vi "CreateLogFile.vi"(0 "Buffers in":T1={"Channels"=[], "PosttriggerBuffer"=refnum, "PretriggerBuffer"=refnum, "BlockSizePerChannel"=0, " logging semaphore"=refnum, "Log refnum"=refnum, "snapshotBuffer"=refnum, "logDirectory"=path "", "logPrefix"="", "decimation factor"=1, "max files"=0, "SampleRate"=0.0}, 11 "error in (no error)":errorcluster) -> (4 "Buffers out":T1={"Channels"=[], "PosttriggerBuffer"=refnum, "PretriggerBuffer"=refnum, "BlockSizePerChannel"=0, " logging semaphore"=refnum, "Log refnum"=refnum, "snapshotBuffer"=refnum, "logDirectory"=path "", "logPrefix"="", "decimation factor"=1, "max files"=0, "SampleRate"=0.0}, 15 "error out":errorcluster)   [LabVIEW 2017, in "BufferLogging.lvlib"]
uses:
  BufferLogging.lvlib
  Buffers.ctl
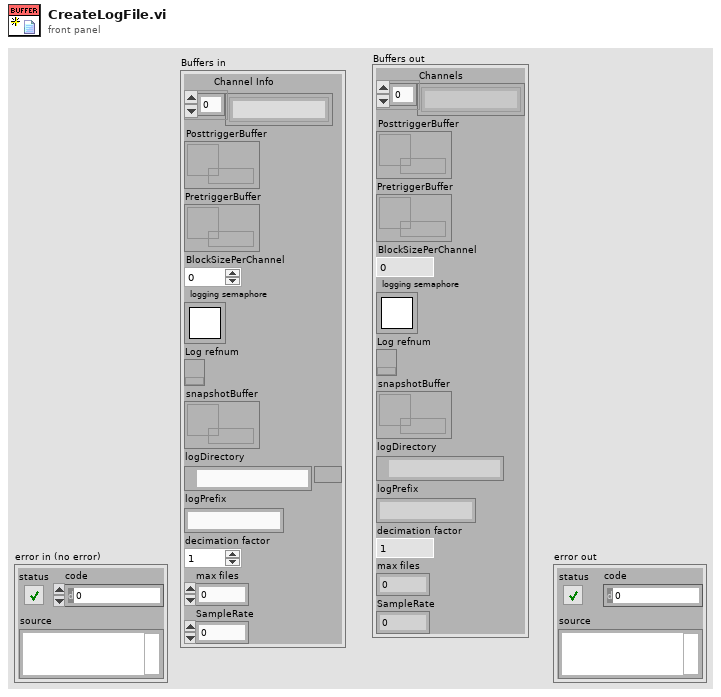
[diagram p1: front panel]
types:
  T1 = typedef "BufferLogging.lvlib/Buffers.ctl" = cluster{"Channels":string[], "PosttriggerBuffer":refnum<queue>, "PretriggerBuffer":refnum<queue>, "BlockSizePerChannel":i32, " logging semaphore":T2, "Log refnum":refnum<k34>, "snapshotBuffer":refnum<data-value>, "logDirectory":path, "logPrefix":string, "decimation factor":i32, "max files":i32, "SampleRate":dbl}
  T2 = typedef "Semaphore RefNum" = refnum<k1>
  T3 = enum16{"open", "open or create", "create or replace", "create", "open (read-only)"}
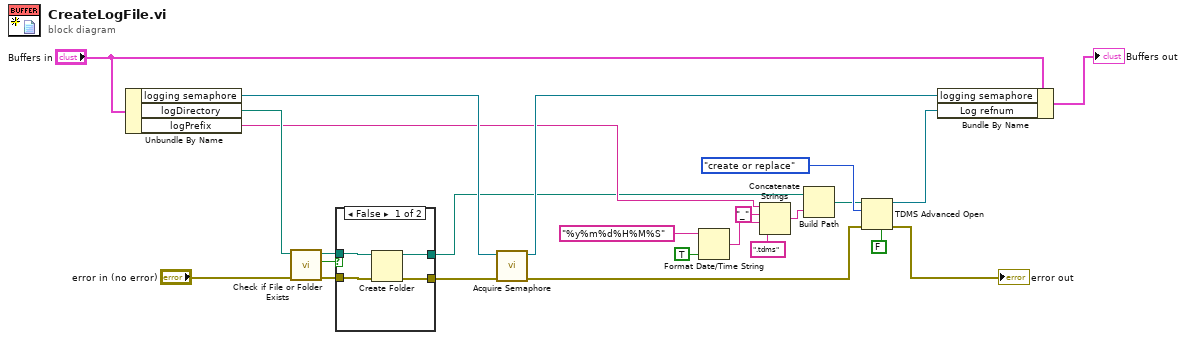
[diagram p0: block diagram]
diagram:
  n1 = Unbundle By Name("Buffers in") -> ("logging semaphore"=w15:T2, "logDirectory"=w3:path, "logPrefix"=w2:string)
  n2 = call <vilib>:"Check if File or Folder Exists.vi"("error in (no error)"="error in (no error)", "path"=w3) -> ("error out"=w6:errorcluster, "file or folder exists?"=w8:bool, "dup path"=w7:path)  [unwired: 7 in]
  n3 = case shown="False" w8 {
    tunnel: w7 -> [w27 w30]
    tunnel: w6 -> [w28 w29]
    tunnel: [w26 w30] -> w1
    tunnel: [w25 w29] -> w4
    frame False {
      n4 = Create Folder(path (use dialog)=w27, error in=w28) -> (created path=w26:path, error out=w25:errorcluster)  [unwired: 1 in, 1 out]
    }
    frame True {
    }
  }
  n5 = call <vilib>:"Acquire Semaphore.vi"("error in (no error)"=w4, "semaphore"=w15) -> ("error out"=w14:errorcluster, "semaphore out"=w12:T2)  [unwired: 3 in, 1 out]
  n6 = Format Date/Time String(time format string (%c)="%y%m%d%H%M%S", UTC format=TRUE) -> (date/time string=w18:string)  [unwired: 1 in]
  n7 = Concatenate Strings(w2, "_" ("string"), w18, ".tdms" ("string")) -> (w21:string)
  n8 = Build Path(base path=w1, name or relative path=w21) -> (appended path=w22:path)
  n9 = TDMS Advanced Open(4:FALSE ("enable asynchronous? (T)"), 8:w14, 10:T3."create or replace" ("operation (0:open)"), 11:w22) -> (0:→"error out":errorcluster, 3:w11:refnum<k34>)  [unwired: 1 in, 1 out]
  n10 = Bundle By Name(cluster="Buffers in", "logging semaphore"=w12, "Log refnum"=w11) -> (→"Buffers out":T1)
